vi "Dialog.MassStepGeneration.vi"(8 "error in (no error)":errorcluster, 11 "State Variables":T1={"Aliases.All"=[], "Aliases.Outputs"=[], "UI.Sequence#ofColumns"=0, "SysDef.Path"=path "", "UI.SequenceRef"=refnum, "UI.StepInformationRef"=refnum, "UI.AbortRef"=refnum, "UI.GraphRef"=refnum, "UI.ViewRef"=refnum, "UI.IterationsRef"=refnum, "UI.IterationInformationRef"=refnum, "INI.Settings"={"Build Location"=path "C:/Simple Sequence Editor/SequenceRepo", "LoggingLocation"=path ""}}) -> (0 "error out":errorcluster)   [LabVIEW 2013, in "Simple Sequence Tools - Editor.lvlib"]
uses:
  Simple Sequence Tools - Editor.lvlib
  Types/StateVariables.ctl
  Shared/Types/ChannelProperties.ctl
  Shared/Types/INI.Settings
  Shared/Simple Sequence Tools - Shared.lvlib
panel:
  in  "Cancel":bool
  in  "OK":bool
  in  "Starting Step Index":u16 max=0
  in  "Value Increment":dbl
  in  "# of Step":u16=1
  in  "Base Step":string(combo)="Step (Value)"
  in  "Alias":string(combo)
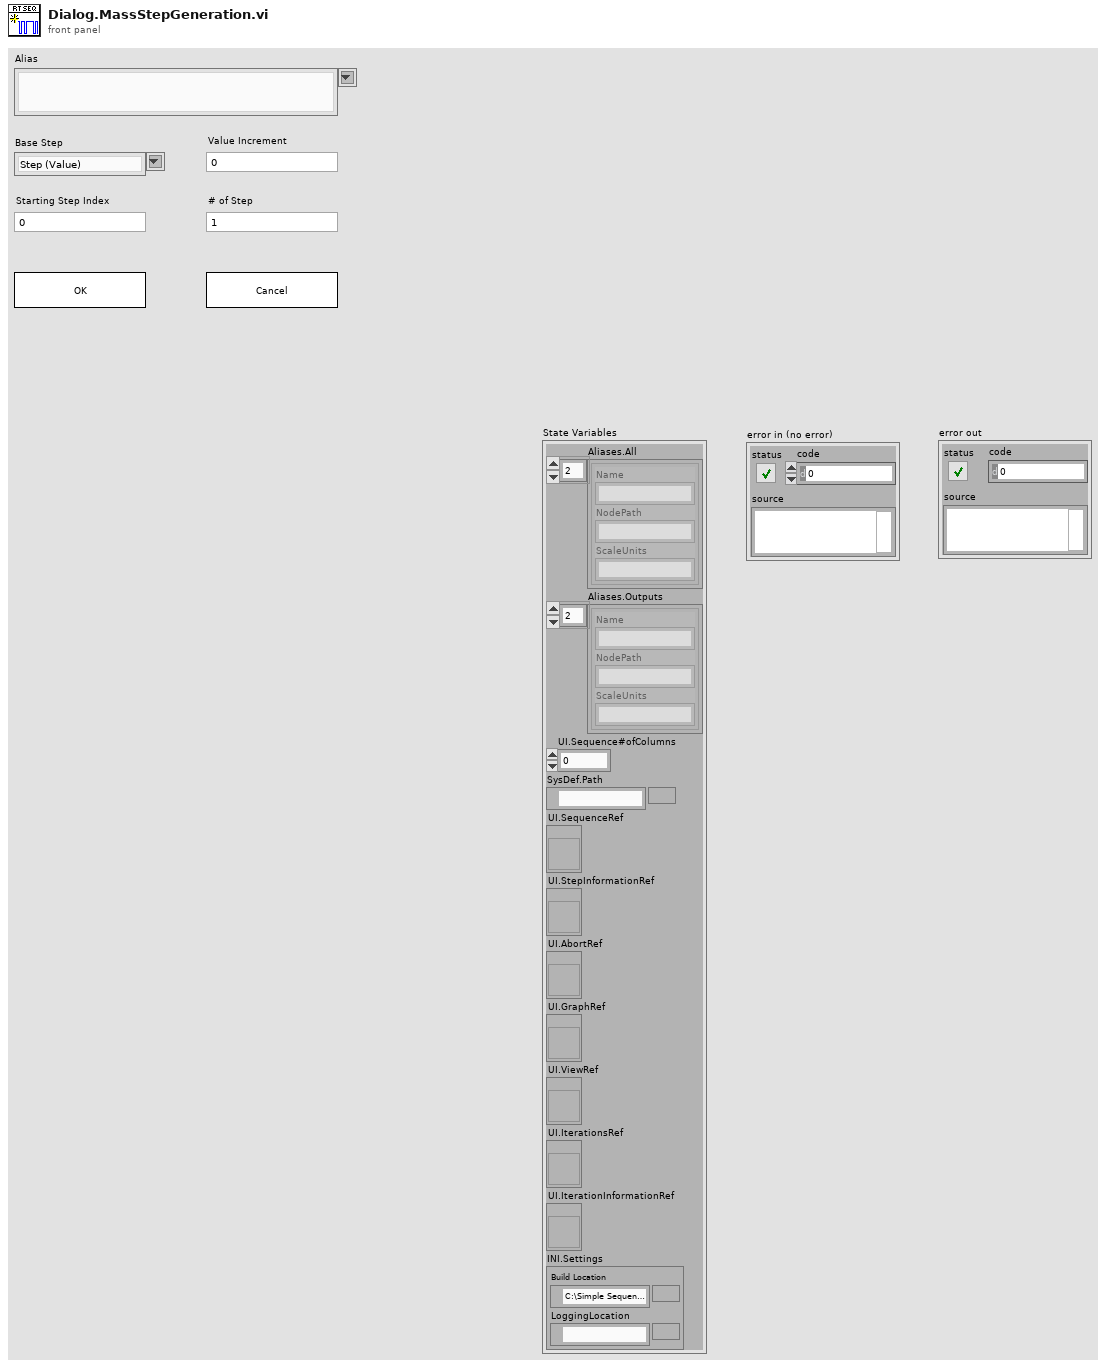
[diagram p1: front panel]
types:
  T1 = typedef "Simple Sequence Tools - Editor.lvlib/StateVariables.ctl" = cluster{"Aliases.All":T2[], "Aliases.Outputs":T2[], "UI.Sequence#ofColumns":i32, "SysDef.Path":path, "UI.SequenceRef":refnum<vi>, "UI.StepInformationRef":refnum<vi>, "UI.AbortRef":refnum<vi>, "UI.GraphRef":refnum<vi>, "UI.ViewRef":refnum<vi>, "UI.IterationsRef":refnum<vi>, "UI.IterationInformationRef":refnum<vi>, "INI.Settings":T3}
  T2 = typedef "Simple Sequence Tools - Shared.lvlib/ChannelProperties.ctl" = cluster{"Name":string, "NodePath":string, "ScaleUnits":string}
  T3 = typedef "Simple Sequence Tools - Shared.lvlib/INI.Settings" = cluster{"Build Location":path, "LoggingLocation":path}
  T4 = enum8{"Enabled", "Disabled", "Disabled and Grayed Out"}
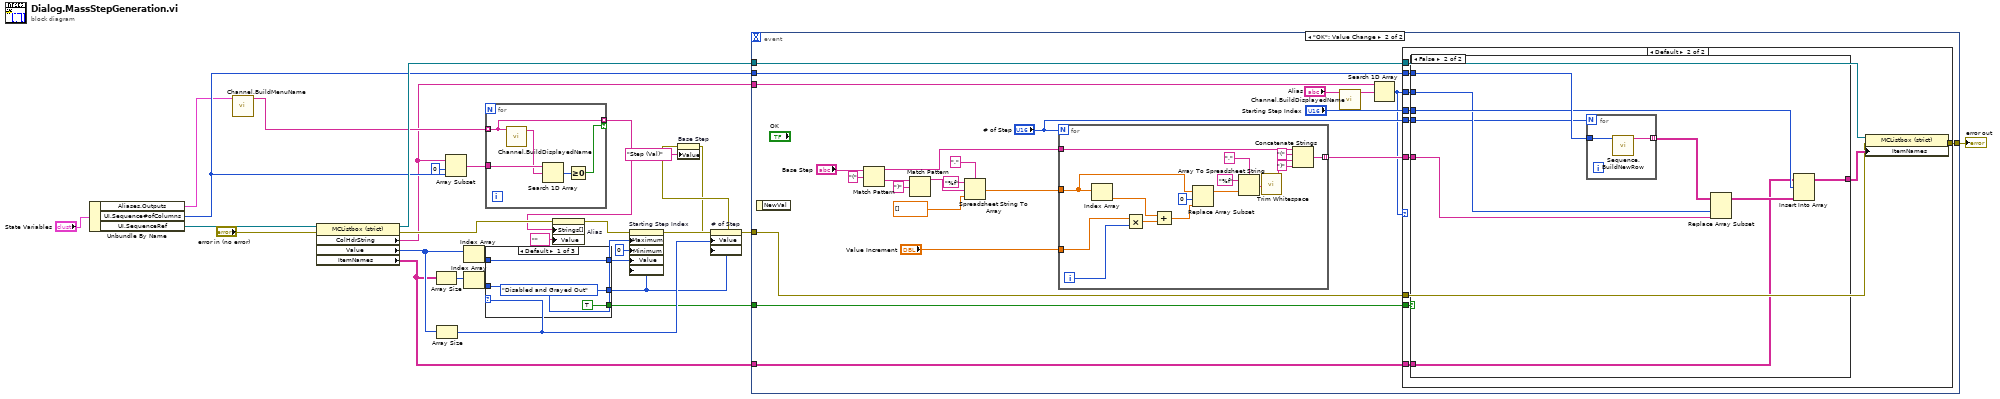
[diagram p0: block diagram]
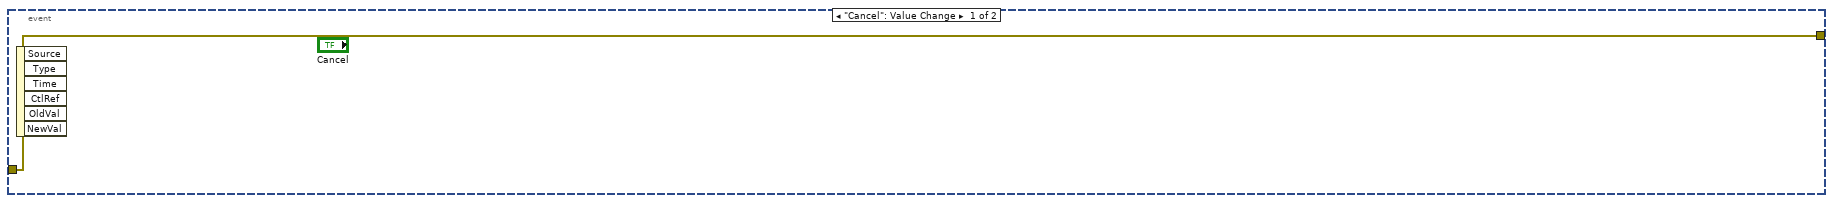
[diagram p2: hidden frame]
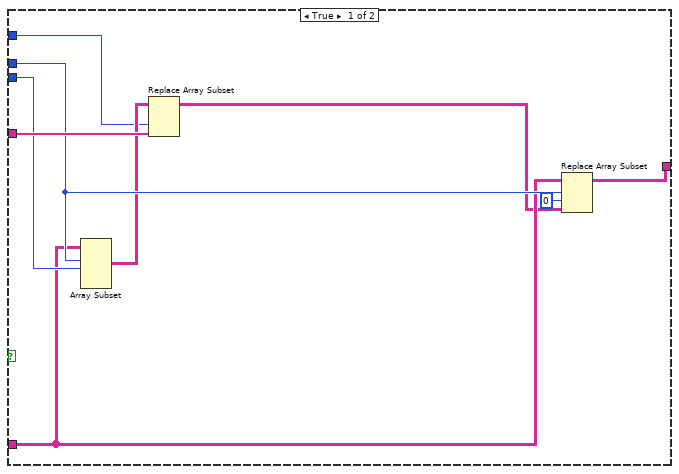
[diagram p4: hidden frame]
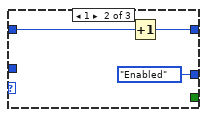
[diagram p5: hidden frame]
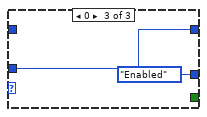
[diagram p6: hidden frame]
diagram:
  n1 = Unbundle By Name("State Variables") -> ("Aliases.Outputs"=w10:T2[], "UI.Sequence#ofColumns"=w18:i32, "UI.SequenceRef"=w28:refnum<vi>)
  n2 = call "Channel.BuildMenuName.vi"("Aliases"=w10) -> ("Aliases Array"=w9:string[])  [unwired: 10 in]
  n3 = property class="MCListbox (strict)"(reference=w28, error in="error in (no error)") -> (reference out=w20:refnum<vi>, error out=w16:errorcluster, "ColHdrString"=w8:string[], "Value"=w22:i32[], "ItemNames"=w21:string[][])
  n4 = Array Size(array=w21) -> (size(s)=w26:i32[])
  n5 = Array Size(array=w22) -> (size(s)=w14:i32)
  n6 = Array Subset(array=w8, index=0, length=w18) -> (w7:string[])
  n7 = Index Array(array=w22) -> (element=w27:i32)  [unwired: 1 in]
  n8 = Index Array(array=w26) -> (element=w25:i32)  [unwired: 1 in]
  n9 = for {
    tunnel: w9 -> [w32] mode=indexing
    tunnel: w7 -> [w34]
    tunnel: [w32] -> w6 mode=indexing if=w30
    n10 = call "Channel.BuildDisplayedName.vi"("Path"=w32) -> ("Formated Path"=w33:string)  [unwired: 10 in]
    n11 = Search 1D Array(1D array=w34, element=w33) -> (index of element=w31:i32)  [unwired: 1 in]
    n12 = Greater Or Equal To 0?(x=w31) -> (x >= 0?=w30:bool)
  }
  n13 = case shown="Default" w14 {
    tunnel: [w37 w39 w42] -> w23
    tunnel: w27 -> [w37 w40 _]
    tunnel: w25 -> [_ _ w42]
    tunnel: [T4."Disabled and Grayed Out" ("Disabled") T4."Enabled" ("Disabled") T4."Enabled" ("Disabled")] -> w12
    tunnel: [TRUE _ _] -> w11
    frame Default {
    }
    frame 1 {
      n14 = Increment(x=w40) -> (x+1=w39:i32)
    }
    frame 0 {
    }
  }
  n15 = property on="Alias" class="CmbBox"(error in=w16, "Strings[]"=w6, "Value"="" ("Alias")) -> (error out=w15:errorcluster)  [unwired: 1 in, 1 out]
  n16 = property on="Starting Step Index" class="DigNum (strict)"(error in=w15, "Maximum"=w25, "Minimum"=0, "Value"=w23, "DisabledEnum"=w12) -> (error out=w13:errorcluster)  [unwired: 1 in, 1 out]
  n17 = property on="# of Step" class="DigNum (strict)"(error in=w13, "Value"=w14, "DisabledEnum"=w12) -> (error out=w3:errorcluster)  [unwired: 1 in, 1 out]
  n18 = property on="Base Step" class="CmbBox"(error in=w3, "Value"="Step (Val)" ("Base Step")) -> (error out=w2:errorcluster)  [unwired: 1 in, 1 out]
  n19 = event shown="[1] \"OK\": Value Change" {
    selector: _ -> [_ _]
    dyn-events: _ -> [_ _]
    timeout: _ -> [_ _]
    tunnel: w2 -> [w43 w47]
    tunnel: w8 -> [_ w55]
    tunnel: w21 -> [_ w52]
    tunnel: w18 -> [_ w53]
    tunnel: w20 -> [_ w49]
    tunnel: [w43 w46] -> w19
    tunnel: w11 -> [_ w45]
    event "Cancel": Value Change {
      n20 = event-data() -> ()  [unwired: 1 in, 6 out]
    }
    event "OK": Value Change {
      n21 = event-data() -> ()  [unwired: 1 in, 1 out]
      n22 = Match Pattern(string="Base Step", regular expression="(") -> (before substring=w57:string, after substring=w65:string)  [unwired: 1 in, 2 out]
      n23 = Match Pattern(string=w65, regular expression=")") -> (before substring=w63:string)  [unwired: 1 in, 3 out]
      n24 = Spreadsheet String To Array(delimiter (Tab)=",", format string="%f", spreadsheet string=w63, array type (2D Dbl)=dbl[] []) -> (array=w59:dbl[])
      n25 = for {
        N: "# of Step" -> [_]
        tunnel: w59 -> [w111]
        tunnel: "Value Increment" -> [w115]
        tunnel: w57 -> [w105]
        tunnel: [w101] -> w48 mode=indexing
        i -> [w114]
        n26 = Index Array(array=w111) -> (element=w112:dbl)  [unwired: 1 in]
        n27 = Multiply(x=w115, y=w114) -> (x*y=w113:dbl)
        n28 = Add(x=w112, y=w113) -> (x+y=w109:dbl)
        n29 = Replace Array Subset(array=w111, new element=w109, index=0) -> (w108:dbl[])
        n30 = Array To Spreadsheet String(delimiter (Tab)=",", array=w108, 3:"%f" ("format string")) -> (spreadsheet string=w103:string)
        n31 = call <vilib>:"Trim Whitespace.vi"("string"=w103) -> ("trimmed string"=w100:string)  [unwired: 1 in]
        n32 = Concatenate Strings(w105, "(" ("string"), w100, ")" ("string")) -> (w101:string)
      }
      n33 = call "Channel.BuildDisplayedName.vi"("Path"="Alias") -> ("Formated Path"=w54:string)  [unwired: 10 in]
      n34 = Search 1D Array(1D array=w55, element=w54) -> (index of element=w44:i32)  [unwired: 1 in]
      n35 = case shown="Default" w44 {
        tunnel: w53 -> [_ w79]
        tunnel: w52 -> [_ w78]
        tunnel: "# of Step" -> [_ w77]
        tunnel: "Starting Step Index" -> [_ w76]
        tunnel: w49 -> [_ w74]
        tunnel: w44 -> [_ w73]
        tunnel: w48 -> [_ w72]
        tunnel: w47 -> [w68 w71]
        tunnel: [w68 w70] -> w46
        tunnel: w45 -> [_ w69]
        frame -1 {
        }
        frame Default {
          n36 = case shown="False" w69 {
            tunnel: w79 -> [_ w97]
            tunnel: w78 -> [w83 w89]
            tunnel: w77 -> [w85 w92]
            tunnel: w76 -> [w86 w96]
            tunnel: [w88 w95] -> w75
            tunnel: w73 -> [w81 w93]
            tunnel: w72 -> [w87 w90]
            frame True {
              n37 = Array Subset(array=w83, index (row)=w86, length (row)=w85) -> (w84:string[][])  [unwired: 2 in]
              n38 = Replace Array Subset(array=w84, new element=w87, index (col)=w81) -> (w82:string[][])  [unwired: 1 in]
              n39 = Replace Array Subset(array=w83, new element=w82, index (row)=w86, index (col)=0 ("disabled index (col)")) -> (w88:string[][])
            }
            frame False {
              n40 = for {
                N: w92 -> [_]
                tunnel: w97 -> [w99]
                tunnel: [w98] -> w91 mode=indexing
                n41 = call "Sequence.BuildNewRow.vi"("UI.Sequence#ofColumns"=w99) -> ("New Array"=w98:string[])  [unwired: 10 in]
              }
              n42 = Replace Array Subset(array=w91, new element=w90, index (col)=w93) -> (w94:string[][])  [unwired: 1 in]
              n43 = Insert Into Array(array=w89, index (row)=w96, new element=w94) -> (w95:string[][])  [unwired: 1 in]
            }
          }
          n44 = property class="MCListbox (strict)"(reference=w74, error in=w71, "ItemNames"=w75) -> (error out=w70:errorcluster)  [unwired: 1 out]
        }
      }
    }
  }
  "error out" <- w19
